vi "FPGA_SystemGet.vi"() -> (3 "FRC FPGA Ref":T1)   [LabVIEW 2017]
uses:
  <vilib>/Rock Robotics/SystemInterfaces/System/FPGA_SystemFRC FPGA Ref.ctl
  <vilib>/Rock Robotics/SystemInterfaces/System/FPGA_SystemFPGA Ref Global.vi
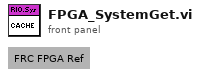
[diagram p1: front panel]
types:
  T1 = typedef "FPGA_SystemFRC FPGA Ref.ctl" = refnum<k20>
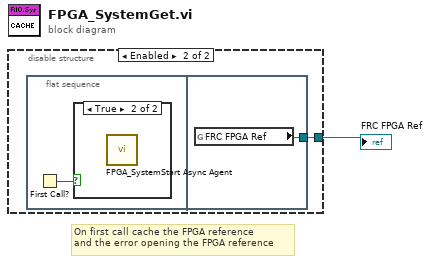
[diagram p0: block diagram]
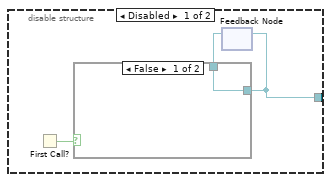
[diagram p2: hidden frame]
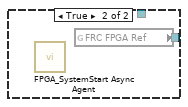
[diagram p3: hidden frame]
diagram:
  # "On first call cache the FPGA reference\nand the error opening the FPGA reference"
  n1 = disable-structure shown="Enabled" {
    disable-tunnel: [w3 w7] -> w1
    frame Disabled {
      n2 = First Call?() -> (First Call?: T/F=w4:bool)
      n3 = feedback #1() -> (w2:T1)  [unwired: 1 in]
      n4 = case shown="False" w4 {
        tunnel: [w5 w6] -> w3
        tunnel: w2 -> [w5 _]
        frame False {
        }
        frame True {
          n5 = call <vilib>:"FPGA_SystemStart Async Agent.vi"() -> ()  [unwired: 2 in, 10 out]
          n6 = global read "FPGA_SystemFPGA Ref Global.vi" "FRC FPGA Ref"() -> (w6:T1)
        }
      }
      n7 = feedback-in #1(w3) -> ()
    }
    frame Enabled {
      n8 = flat-sequence {
        tunnel: [w9] -> w7
        frame #0 {
          n9 = First Call?() -> (First Call?: T/F=w8:bool)
          n10 = case shown="True" w8 {
            frame False {
            }
            frame True {
              n11 = call <vilib>:"FPGA_SystemStart Async Agent.vi"() -> ()  [unwired: 2 in, 10 out]
            }
          }
        }
        frame #1 {
          n12 = global read "FPGA_SystemFPGA Ref Global.vi" "FRC FPGA Ref"() -> (w9:T1)
        }
      }
    }
  }
  "FRC FPGA Ref" <- w1
